vi "Peaks Scatter Plot.vi"(0 "Host Plot Controls":T2={"refresh"=FALSE, "PMTs for Host"={"Sa"=1, "Sb"=0, "g-factor"=1}, "Peaks"={"# bins"=100, "min"=0.0, "max"=10.0}, "Averages"={"# bins"=100, "max"=10.0, "min"=0.0}, "Durations"={"# bins"=100, "max"=10.0, "min"=0.0}, "FP-FPGA"={"# bins"=100, "max"=50.0, "min"=0.0}, "FP-Host"={"# bins"=100, "max"=12.0, "min"=8.0}}, 7 "peaks data":T1, 11 "?":cluster{i32[], i32[]}) -> (1 "number points plotted":i32, 2 "FP maxes":cluster{"Max1":dbl[], "Max1":dbl[]}(graph), 3 "FP Averages":cluster{"Max1":dbl[], "Max1":dbl[]}(graph), 4 "scatter maxes":cluster{"Max1":dbl[], "Max1":dbl[]}[](graph), 5 "Sorted and Detected Sums":cluster{"Max1":dbl[], dbl[]}[](graph), 6 "scatter averages":cluster{"Sum1":dbl[], "Sum1":dbl[]}[](graph), 8 "Host_H(FPm) vs. FPm":cluster{"Axis":dbl[], i32[]}(graph), 9 "Sorted and Detected Maxes":cluster{"Max1":dbl[], dbl[]}[](graph), 10 "Host_H(FPa) vs. FPa":cluster{"Axis":dbl[], i32[]}(graph), 13 "Max of PMTa vs. Tin":cluster{"ave1":dbl[], "ave1":dbl[]}(graph), 14 "tin v tout":cluster{"Max1":dbl[], "Max1":dbl[]}(graph), 15 "?":cluster{i32[], i32[]})   [LabVIEW 2009]
uses:
  <vilib>/Analysis/NI_AALPro.lvlib
  <vilib>/Analysis/NI_AALBase.lvlib
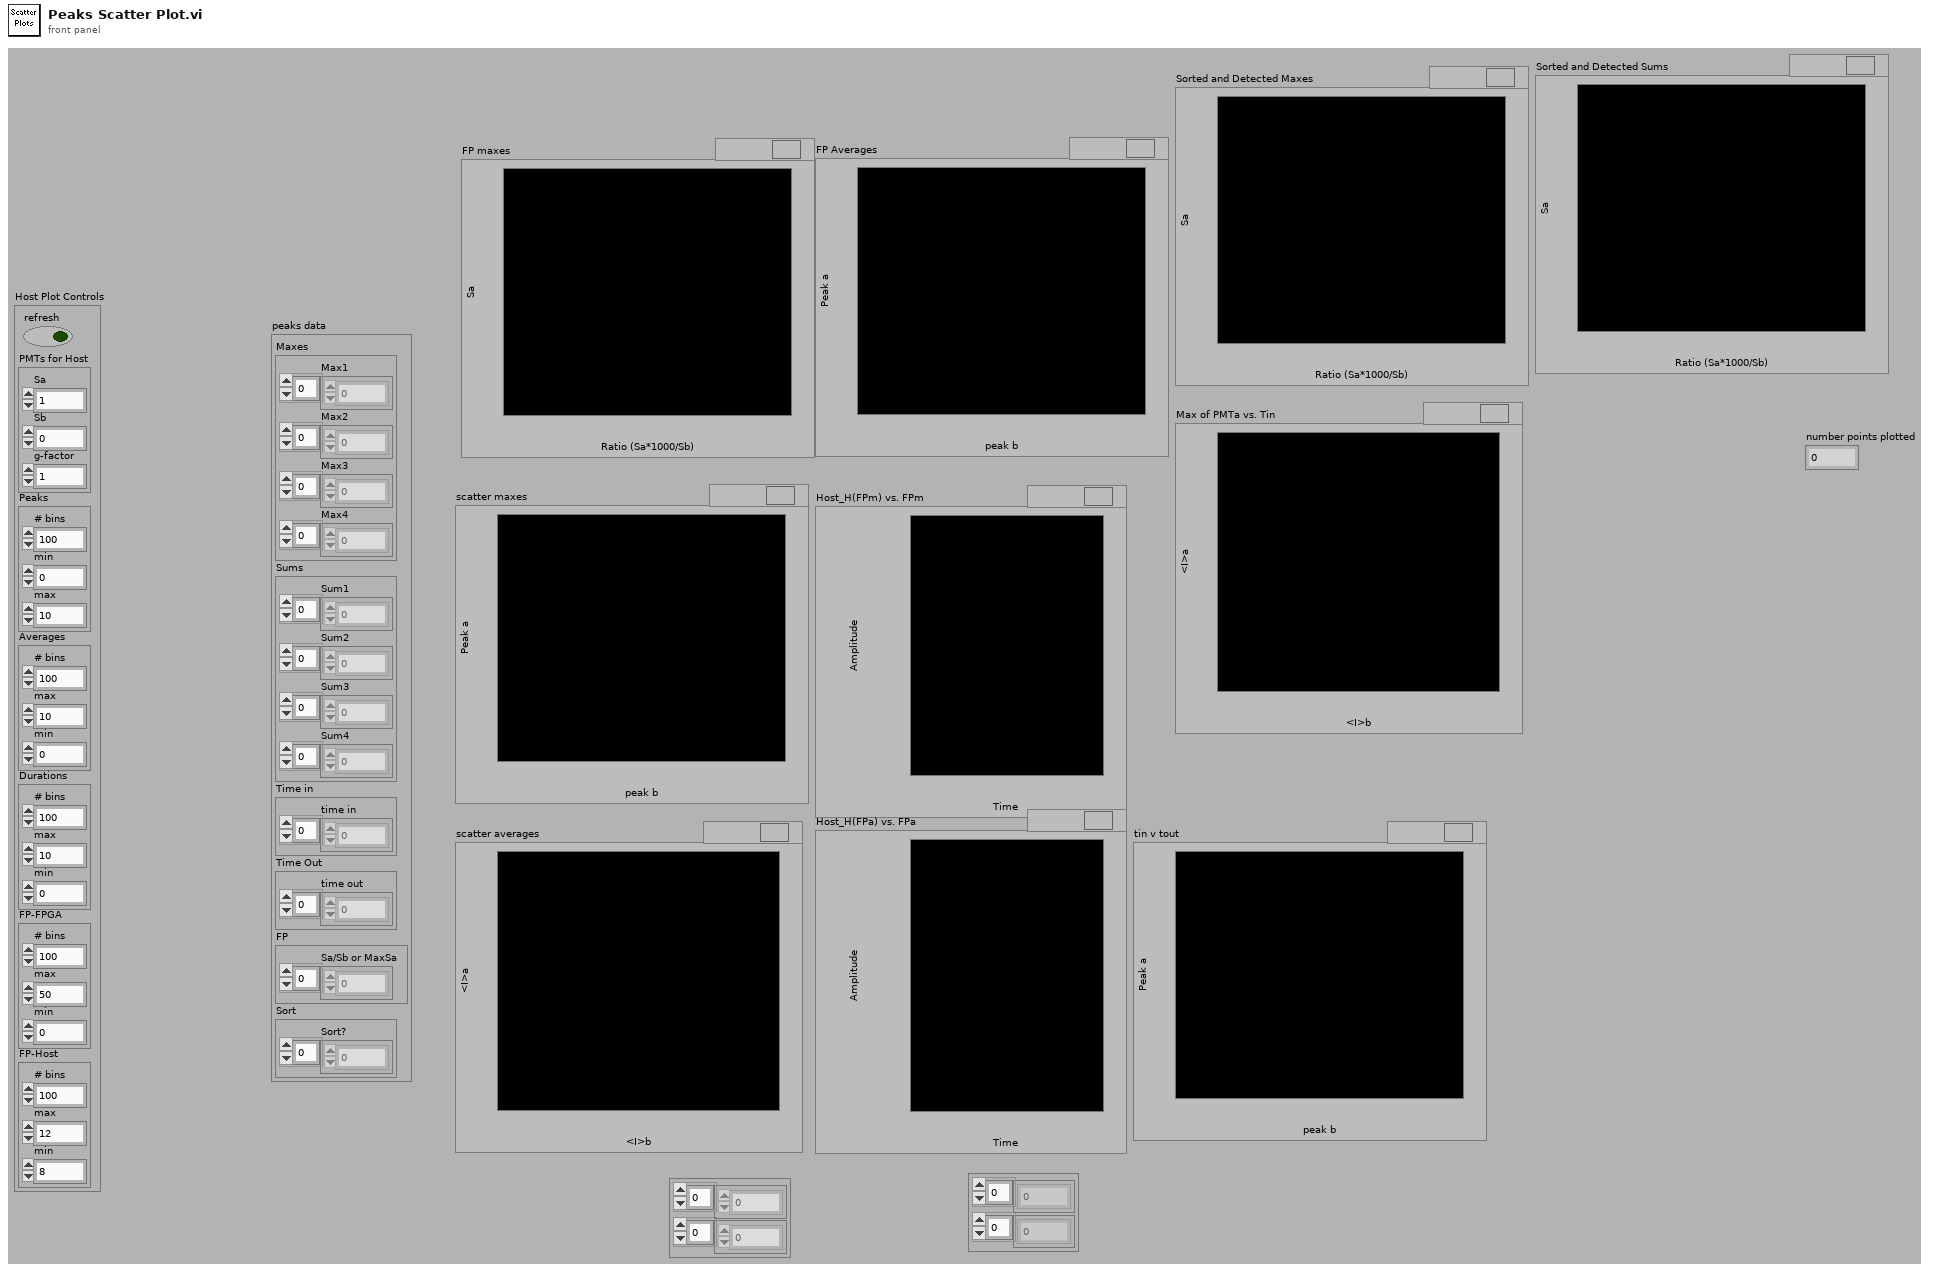
[diagram p1: front panel]
types:
  T1 = cluster{"Maxes":cluster{"Max1":dbl[], "Max2":dbl[], "Max3":dbl[], "Max4":dbl[]}, "Sums":cluster{"Sum1":dbl[], "Sum2":dbl[], "Sum3":dbl[], "Sum4":dbl[]}, "Time in":cluster{"time in":dbl[]}, "Time Out":cluster{"time out":dbl[]}, "FP":cluster{"Sa/Sb or MaxSa":dbl[]}, "Sort":cluster{"Sort?":dbl[]}}
  T2 = cluster{"refresh":bool, "PMTs for Host":cluster{"Sa":i8, "Sb":i8, "g-factor":i32}, "Peaks":cluster{"# bins":i32, "min":dbl, "max":dbl}, "Averages":cluster{"# bins":i32, "max":dbl, "min":dbl}, "Durations":cluster{"# bins":i32, "max":dbl, "min":dbl}, "FP-FPGA":cluster{"# bins":i32, "max":dbl, "min":dbl}, "FP-Host":cluster{"# bins":i32, "max":dbl, "min":dbl}}
  T3 = cluster{"Max1":dbl[], "Max2":dbl[], "Max3":dbl[], "Max4":dbl[]}
  T4 = cluster{"Sum1":dbl[], "Sum2":dbl[], "Sum3":dbl[], "Sum4":dbl[]}
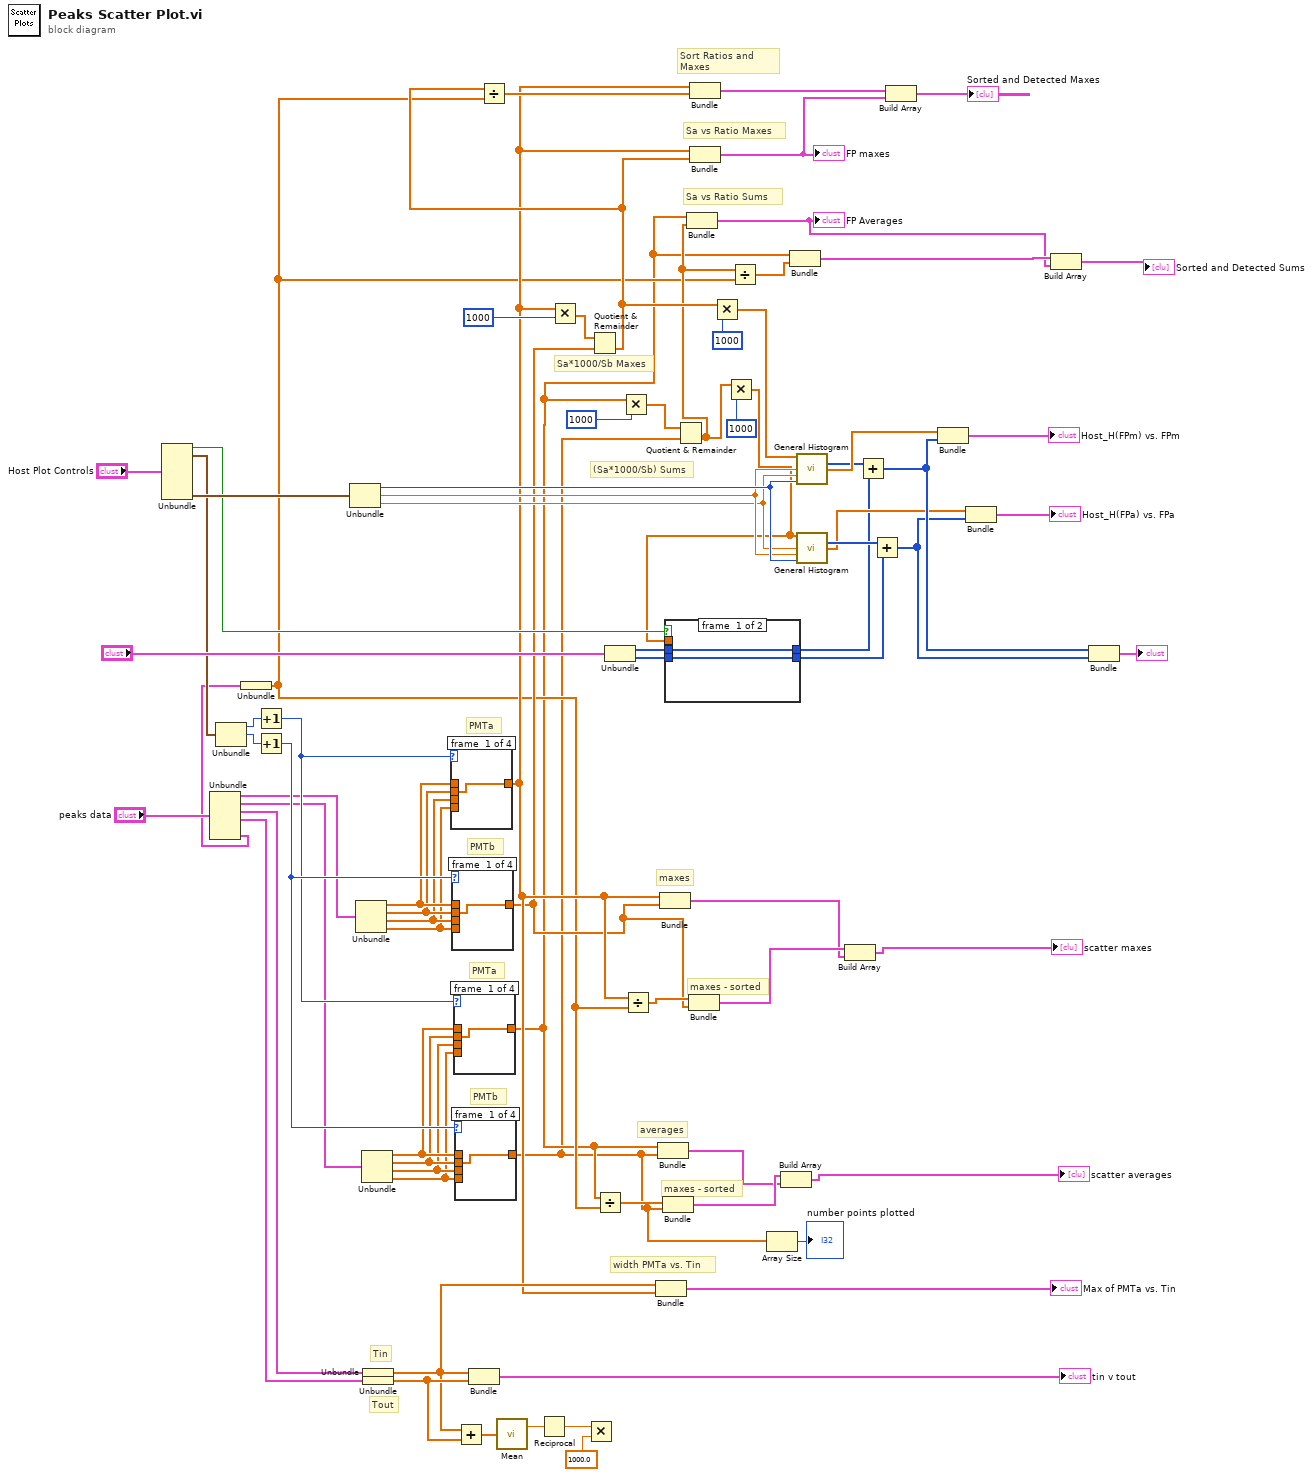
[diagram p0: block diagram]
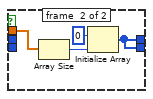
[diagram p2: hidden frame]
diagram:
  # "maxes - sorted"
  # "maxes - sorted"
  # "Sort Ratios and Maxes"
  # "width PMTa vs. Tin"
  # "Tout"
  # "Tin"
  # "Sa vs Ratio Sums"
  # "Sa vs Ratio Maxes"
  # "(Sa*1000/Sb) Sums"
  # "Sa*1000/Sb Maxes"
  # "averages"
  # "maxes"
  # "PMTb"
  # "PMTa"
  # "PMTb"
  # "PMTa"
  n1 = Unbundle("Host Plot Controls") -> ("refresh"=w51:bool, "PMTs for Host"=w31:cluster{"Sa":i8, "Sb":i8, "g-factor":i32}, "FP-Host"=w57:cluster{"# bins":i32, "max":dbl, "min":dbl})  [unwired: 4 out]
  n2 = Unbundle("peaks data") -> ("Maxes"=w65:T3, "Sums"=w64:T4, "Time in"=w63:cluster{"time in":dbl[]}, "Time Out"=w62:cluster{"time out":dbl[]}, "Sort"=w25:cluster{"Sort?":dbl[]})  [unwired: 1 out]
  n3 = Unbundle(w31) -> ("Sa"=w53:i8, "Sb"=w52:i8)  [unwired: 1 out]
  n4 = Unbundle(w25) -> ("Sort?"=w9:dbl[])
  n5 = Increment(x=w53) -> (x+1=w66:i8)
  n6 = Increment(x=w52) -> (x+1=w67:i8)
  n7 = Unbundle(w57) -> ("# bins"=w56:i32, "max"=w55:dbl, "min"=w54:dbl)
  n8 = Unbundle(w65) -> ("Max1"=w46:dbl[], "Max2"=w45:dbl[], "Max3"=w44:dbl[], "Max4"=w43:dbl[])
  n9 = Unbundle(w64) -> ("Sum1"=w42:dbl[], "Sum2"=w41:dbl[], "Sum3"=w40:dbl[], "Sum4"=w39:dbl[])
  n10 = Unbundle(w63) -> ("time in"=w35:dbl[])
  n11 = Unbundle(w62) -> ("time out"=w36:dbl[])
  n12 = case shown="1, Default" w66 {
    tunnel: w46 -> [_ _ _ w83]
    tunnel: w45 -> [w80 _ _ _]
    tunnel: w44 -> [_ w81 _ _]
    tunnel: w43 -> [_ _ w82 _]
    tunnel: [w80 w81 w82 w83] -> w13
    frame #0 {
    }
    frame #1 {
    }
    frame #2 {
    }
    frame #3 {
    }
  }
  n13 = case shown="1, Default" w67 {
    tunnel: w46 -> [_ _ _ w87]
    tunnel: w45 -> [w84 _ _ _]
    tunnel: w44 -> [_ w85 _ _]
    tunnel: w43 -> [_ _ w86 _]
    tunnel: [w84 w85 w86 w87] -> w12
    frame #0 {
    }
    frame #1 {
    }
    frame #2 {
    }
    frame #3 {
    }
  }
  n14 = case shown="1, Default" w66 {
    tunnel: w42 -> [_ _ _ w91]
    tunnel: w41 -> [w88 _ _ _]
    tunnel: w40 -> [_ w89 _ _]
    tunnel: w39 -> [_ _ w90 _]
    tunnel: [w88 w89 w90 w91] -> w8
    frame #0 {
    }
    frame #1 {
    }
    frame #2 {
    }
    frame #3 {
    }
  }
  n15 = case shown="4" w67 {
    tunnel: w42 -> [_ _ _ w95]
    tunnel: w41 -> [w92 _ _ _]
    tunnel: w40 -> [_ w93 _ _]
    tunnel: w39 -> [_ _ w94 _]
    tunnel: [w92 w93 w94 w95] -> w2
    frame #0 {
    }
    frame #1 {
    }
    frame #2 {
    }
    frame #3 {
    }
  }
  n16 = Add(x=w35, y=w36) -> (x+y=w60:dbl[])
  n17 = Bundle("time in"=w35, "time out"=w36) -> (→"tin v tout":cluster{"time in":dbl[], "time out":dbl[]})  [unwired: 1 in]
  n18 = call <vilib>:"Mean.vi"("X"=w60) -> ("mean"=w37:dbl)  [unwired: 1 out]
  n19 = Reciprocal(x=w37) -> (1/x=w59:dbl)
  n20 = Multiply(x=w13, y=1000) -> (x*y=w29:dbl[])
  n21 = Multiply(x=w59, y=1000.0) -> ()  [unwired: 1 out]
  n22 = Quotient & Remainder(x=w29, y=w12) -> (floor(x/y)=w23:dbl[])  [unwired: 1 out]
  n23 = Divide(x=w23, y=w9) -> (x/y=w24:dbl[])
  n24 = Divide(x=w8, y=w9) -> (x/y=w10:dbl[])
  n25 = Unbundle("?") -> (w76:i32[], w69:i32[])
  n26 = Multiply(x=w8, y=1000) -> (x*y=w27:dbl[])
  n27 = Divide(x=w13, y=w9) -> (x/y=w14:dbl[])
  n28 = Bundle("time in"=w35, "Max1"=w13) -> (→"Max of PMTa vs. Tin":cluster{"time in":dbl[], "Max1":dbl[]})  [unwired: 1 in]
  n29 = Bundle("Sum1"=w8, "Sum1"=w2) -> (w3:cluster{"Sum1":dbl[], "Sum1":dbl[]})  [unwired: 1 in]
  n30 = Bundle("Max1"=w13, "Max1"=w12) -> (w5:cluster{"Max1":dbl[], "Max1":dbl[]})  [unwired: 1 in]
  n31 = Bundle(w10, "Sum1"=w2) -> (w4:cluster{dbl[], "Sum1":dbl[]})  [unwired: 1 in]
  n32 = Quotient & Remainder(x=w27, y=w2) -> (floor(x/y)=w19:dbl[])  [unwired: 1 out]
  n33 = Bundle("Sum1"=w8, w19) -> (w15:cluster{"Sum1":dbl[], dbl[]})  [unwired: 1 in]
  "FP Averages" <- w15
  n34 = Bundle(w14, "Max1"=w12) -> (w6:cluster{dbl[], "Max1":dbl[]})  [unwired: 1 in]
  n35 = Bundle("Max1"=w13, w24) -> (w21:cluster{"Max1":dbl[], dbl[]})  [unwired: 1 in]
  n36 = Bundle("Max1"=w13, w23) -> (w20:cluster{"Max1":dbl[], dbl[]})  [unwired: 1 in]
  "FP maxes" <- w20
  n37 = Multiply(x=w23, y=1000) -> (x*y=w48:dbl[])
  n38 = Multiply(x=w19, y=1000) -> (x*y=w26:dbl[])
  n39 = case shown="False" w51 {
    tunnel: w76 -> [w97 _]
    tunnel: w69 -> [w96 _]
    tunnel: [w97 w100] -> w72
    tunnel: [w96 w100] -> w71
    tunnel: w26 -> [_ w99]
    frame #0 {
    }
    frame #1 {
      n40 = Array Size(array=w99) -> (size(s)=w98:i32)
      n41 = Initialize Array(0, w98) -> (w100:i32[])
    }
  }
  n42 = Divide(x=w19, y=w9) -> (x/y=w18:dbl[])
  n43 = Array Size(array=w2) -> (size(s)=→"number points plotted":i32)
  n44 = Build Array(w4, w3) -> (→"scatter averages":cluster{"Sum1":dbl[], "Sum1":dbl[]}[])
  n45 = Bundle("Sum1"=w8, w18) -> (w17:cluster{"Sum1":dbl[], dbl[]})  [unwired: 1 in]
  n46 = call <vilib>:"General Histogram.vi"("X"=w48, "max"=w55, "min"=w54, "# bins"=w56) -> ("Histogram"=w77:i32[], "Axis"=w78:dbl[])  [unwired: 7 in, 3 out]
  n47 = call <vilib>:"General Histogram.vi"("X"=w26, "max"=w54, "min"=w55, "# bins"=w56) -> ("Histogram"=w74:i32[], "Axis"=w73:dbl[])  [unwired: 7 in, 3 out]
  n48 = Build Array(w6, w5) -> (→"scatter maxes":cluster{"Max1":dbl[], "Max1":dbl[]}[])
  n49 = Add(x=w77, y=w72) -> (x+y=w75:i32[])
  n50 = Add(x=w74, y=w71) -> (x+y=w70:i32[])
  n51 = Build Array(w21, w20) -> (→"Sorted and Detected Maxes":cluster{"Max1":dbl[], dbl[]}[])
  n52 = Bundle("Axis"=w78, w75) -> (→"Host_H(FPm) vs. FPm":cluster{"Axis":dbl[], i32[]})  [unwired: 1 in]
  n53 = Bundle("Axis"=w73, w70) -> (→"Host_H(FPa) vs. FPa":cluster{"Axis":dbl[], i32[]})  [unwired: 1 in]
  n54 = Build Array(w17, w15) -> (→"Sorted and Detected Sums":cluster{"Sum1":dbl[], dbl[]}[])
  n55 = Bundle(w75, w70) -> (→"?":cluster{i32[], i32[]})  [unwired: 1 in]
